vi "txt_to_array.vi"(8 "error in":errorcluster, 11 "file (use dialog)":path) -> (0 "error out":errorcluster, 1 "String":string, 2 "array":i32[][](array[numeric]))   [LabVIEW 2013]
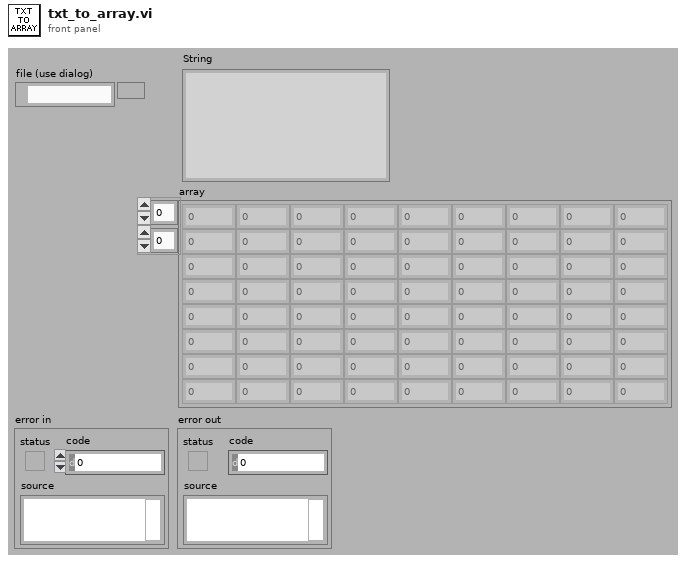
[diagram p1: front panel]
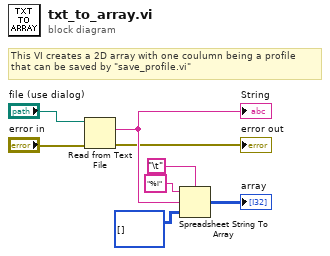
[diagram p0: block diagram]
diagram:
  # "This VI creates a 2D array with one coulumn being a profile\nthat can be saved by \"save_profile.vi\""
  n1 = Read from Text File(file (use dialog)="file (use dialog)", error in="error in") -> (text=w7:string, error out=→"error out":errorcluster)  [unwired: 2 in, 2 out]
  "String" <- w7
  n2 = Spreadsheet String To Array(delimiter (Tab)="\t", format string="%i", spreadsheet string=w7, array type (2D Dbl)=i32[][] []) -> (array=→"array":i32[][])
